vi "ENPH354_A4Q5.vi"() -> ()   [LabVIEW 2020]
uses:
  <vilib>/Utility/file.llb/Read Delimited Spreadsheet (DBL).vi
panel:
  out "Optical Power [mW]":dbl
  out "Conversion Factor [mA/mW]":dbl
  in  "Reduced Responsivity Fitted Data":path
  in  "Corrected WLED Emission":path
  # "ENPH354 Assignment 4 Q5"
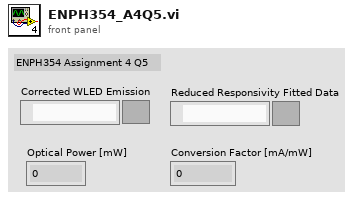
[diagram p1: front panel]
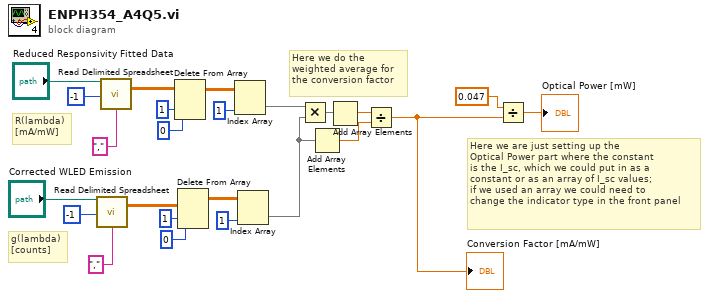
[diagram p0: block diagram]
diagram:
  # "Here we are just setting up the \nOptical Power part where the constant\nis the I_sc, which we could put in as a \nconstant or as an array of I_sc values; \nif we used an array we could need to \nchange the indicator type in the front panel"
  # "Here we do the \nweighted average for \nthe conversion factor"
  # "R(lambda)\n[mA/mW]"
  # "g(lambda)\n[counts]"
  n1 = call-poly <vilib>:"Read Delimited Spreadsheet.vi"("file path (dialog if empty)"="Corrected WLED Emission", "number of rows (all:-1)"=-1, "delimiter (\\t)"="," ("delimiter (\\t)")) -> ("all rows"=w21:dbl[][])  [unwired: 7 in, 5 out]
  n2 = call-poly <vilib>:"Read Delimited Spreadsheet.vi"("file path (dialog if empty)"="Reduced Responsivity Fitted Data", "number of rows (all:-1)"=-1, "delimiter (\\t)"="," ("delimiter (\\t)")) -> ("all rows"=w12:dbl[][])  [unwired: 7 in, 5 out]
  n3 = Delete From Array(array=w12, length=1, index (row)=0) -> (array with subset deleted=w6:dbl[][])  [unwired: 1 in, 1 out]
  n4 = Delete From Array(array=w21, length=1, index (row)=0) -> (array with subset deleted=w7:dbl[][])  [unwired: 1 in, 1 out]
  n5 = Index Array(array=w6, index (col)=1) -> (element=w5:dbl[])  [unwired: 1 in]
  n6 = Index Array(array=w7, index (col)=1) -> (element=w4:dbl[])  [unwired: 1 in]
  n7 = Multiply(x=w5, y=w4) -> (x*y=w10:dbl[])
  n8 = Add Array Elements(numeric array=w4) -> (sum=w8:dbl)
  n9 = Add Array Elements(numeric array=w10) -> (sum=w9:dbl)
  n10 = Divide(x=w9, y=w8) -> (x/y=w3:dbl)
  "Conversion Factor [mA/mW]" <- w3
  n11 = Divide(x=0.047, y=w3) -> (x/y=→"Optical Power [mW]":dbl)
